vi "sub_vi_2.vi"(9 "B":dbl, 10 "X":dbl, 11 "A":dbl) -> (3 "Numeric":dbl)   [LabVIEW 2025]
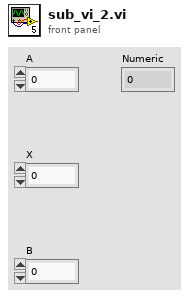
[diagram p1: front panel]
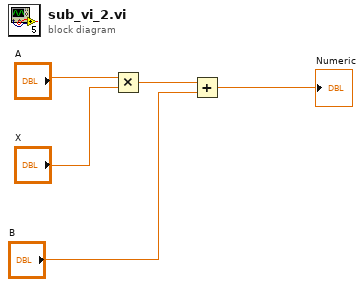
[diagram p0: block diagram]
diagram:
  n1 = Multiply(x="A", y="X") -> (x*y=w2:dbl)
  n2 = Add(x=w2, y="B") -> (x+y=→"Numeric":dbl)
